vi "Init.vi"() -> ()   [LabVIEW 2020]
panel:
  out "Init?":bool
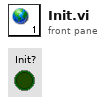
[diagram p1: front panel]
diagram:
